vi "Format_ZCAN_Transmit_Data.vi"(8 "Send_string_data":string, 9 "frame_format":i16, 10 "frame_type":i16, 11 "can_frame.can_id":u32) -> (3 "tagZCAN_Transmit_Data":T1)   [LabVIEW 2020, in "zlgcan.lvlib"]
uses:
  zlgcan.lvlib
  data_type/tagZCAN_Transmit_Data.ctl
  data_type/can_frame.ctl
panel:
  in  "协议":u32(ring) items=["CAN", "CANFD"]
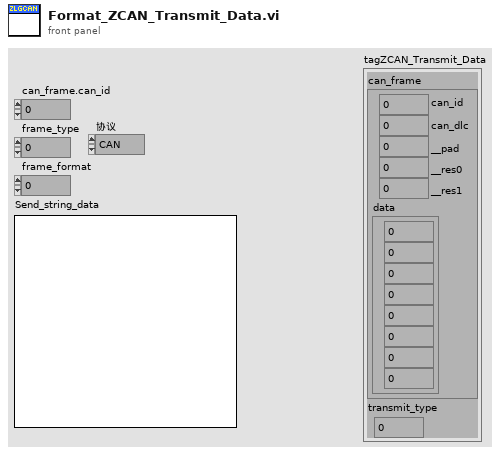
[diagram p1: front panel]
types:
  T1 = typedef "zlgcan.lvlib/tagZCAN_Transmit_Data.ctl" = cluster{"can_frame":T2, "transmit_type":u32}
  T2 = typedef "zlgcan.lvlib/can_frame.ctl" = cluster{"can_id":u32, "can_dlc":u8, "__pad":u8, "__res0":u8, "__res1":u8, "data":cluster{"CAN数据[0]":u8, "CAN数据[1]":u8, "CAN数据[2]":u8, "CAN数据[3]":u8, "CAN数据[4]":u8, "CAN数据[5]":u8, "CAN数据[6]":u8, "CAN数据[7]":u8}}
  T3 = cluster{"[0]":u8, "[1]":u32, "[2]":u32, "[3]":u32, "[4]":u32, "[5]":u32, "[6]":u32, "[7]":u32}
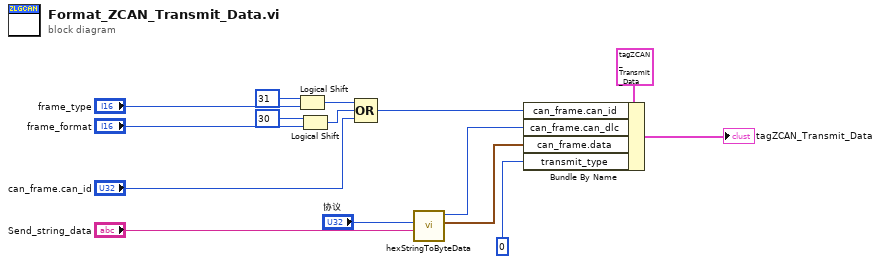
[diagram p0: block diagram]
diagram:
  n1 = Logical Shift(y=i16 31, x="frame_type") -> (x << y=w13:i16)
  n2 = Logical Shift(y=i16 30, x="frame_format") -> (x << y=w10:i16)
  n3 = Compound Arithmetic op=OR ("复合运算")(w13, w10, "can_frame.can_id") -> (w9:u32)
  n4 = call "hexStringToByteData.vi"("数据输入"="Send_string_data", "协议"="协议") -> ("CAN_data"=w8:T3, "字节数"=w5:u8)  [unwired: 6 in, 2 out]
  n5 = Bundle By Name(cluster=T1 {"can_frame"={"can_id"=0, "can_dlc"=0, "__pad"=0, "__res0"=0, "__res1"=0, "data"={"CAN数据[0]"=0, "CAN数据[1]"=0, "CAN数据[2]"=0, "CAN数据[3]"=0, "CAN数据[4]"=0, "CAN数据[5]"=0, "CAN数据[6]"=0, "CAN数据[7]"=0}}, "transmit_type"=0} ("tagZCAN_Transmit_Data.ctl"), "can_frame.can_id"=w9, "can_frame.can_dlc"=w5, "can_frame.data"=w8, "transmit_type"=u32 0) -> (→"tagZCAN_Transmit_Data":T1)
